vi "SetSocketOption.vi"(7 "path override":path, 8 "error in":errorcluster, 9 "value":variant, 10 "Socket option":T1=enum."ZMQ_SWAP", 11 "socket in":u64) -> (0 "error out":errorcluster, 3 "socket out":u64)   [LabVIEW 2025, in "LibZMQ.lvlib"]
uses:
  LibZMQ.lvlib
  ctls/SocketOption.ctl
  errno.vi
  strerror.vi
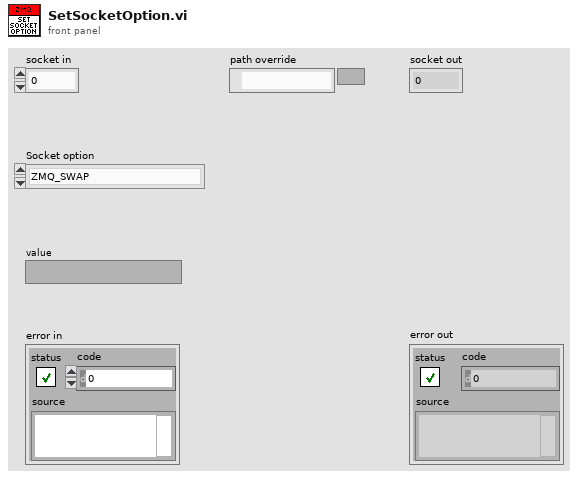
[diagram p1: front panel]
types:
  T1 = typedef "LibZMQ.lvlib/SocketOption.ctl" = enum8{"NONE", "ZMQ_HWM", "<2>", "ZMQ_SWAP", "ZMQ_AFFINITY", "ZMQ_ROUTING_ID", "ZMQ_SUBSCRIBE", "ZMQ_UNSUBSCRIBE", "ZMQ_RATE", "ZMQ_RECOVERY_IVL", "ZMQ_MCAST_LOOP", "ZMQ_SNDBUF", "ZMQ_RCVBUF", "ZMQ_RCVMORE", "ZMQ_FD", "ZMQ_EVENTS", "ZMQ_TYPE", "ZMQ_LINGER", "ZMQ_RECONNECT_IVL", "ZMQ_BACKLOG", "ZMQ_RECOVERY_IVL_MSEC", "ZMQ_RECONNECT_IVL_MAX", "ZMQ_MAXMSGSIZE", "ZMQ_SNDHWM", "ZMQ_RCVHWM", "ZMQ_MULTICAST_HOPS", "<26>", "ZMQ_RCVTIMEO", "ZMQ_SNDTIMEO", "<29>", "<30>", "ZMQ_IPV4ONLY", "ZMQ_LAST_ENDPOINT", "ZMQ_ROUTER_MANDATORY", "ZMQ_TCP_KEEPALIVE", "ZMQ_TCP_KEEPALIVE_CNT", "ZMQ_TCP_KEEPALIVE_IDLE", "ZMQ_TCP_KEEPALIVE_INTVL", "ZMQ_TCP_ACCEPT_FILTER", "ZMQ_IMMEDIATE", "ZMQ_XPUB_VERBOSE", "ZMQ_ROUTER_RAW", "ZMQ_IPV6", "ZMQ_MECHANISM", "ZMQ_PLAIN_SERVER", "ZMQ_PLAIN_USERNAME", "ZMQ_PLAIN_PASSWORD", "ZMQ_CURVE_SERVER", "ZMQ_CURVE_PUBLICKEY", "ZMQ_CURVE_SECRETKEY", "ZMQ_CURVE_SERVERKEY", "ZMQ_PROBE_ROUTER", "ZMQ_REQ_CORRELATE", "ZMQ_REQ_RELAXED", "ZMQ_CONFLATE", "ZMQ_ZAP_DOMAIN", "ZMQ_ROUTER_HANDOVER", "ZMQ_TOS", "ZMQ_IPC_FILTER_PID", "ZMQ_IPC_FILTER_UID", "ZMQ_IPC_FILTER_GID", "ZMQ_CONNECT_ROUTING_ID", "ZMQ_GSSAPI_SERVER", "ZMQ_GSSAPI_PRINCIPAL", "ZMQ_GSSAPI_SERVICE_PRINCIPAL", "ZMQ_GSSAPI_PLAINTEXT", "ZMQ_HANDSHAKE_IVL", "<67>", "ZMQ_SOCKS_PROXY", "ZMQ_XPUB_NODROP", "ZMQ_BLOCKY", "ZMQ_XPUB_MANUAL", "ZMQ_XPUB_WELCOME_MSG", "ZMQ_STREAM_NOTIFY", "ZMQ_INVERT_MATCHING", "ZMQ_HEARTBEAT_IVL", "ZMQ_HEARTBEAT_TTL", "ZMQ_HEARTBEAT_TIMEOUT", "ZMQ_XPUB_VERBOSER", "ZMQ_CONNECT_TIMEOUT", "ZMQ_TCP_MAXRT", "ZMQ_THREAD_SAFE", "<82>", "<83>", "ZMQ_MULTICAST_MAXTPDU", "ZMQ_VMCI_BUFFER_SIZE", "ZMQ_VMCI_BUFFER_MIN_SIZE", "ZMQ_VMCI_BUFFER_MAX_SIZE", "ZMQ_VMCI_CONNECT_TIMEOUT", "ZMQ_USE_FD", "ZMQ_GSSAPI_PRINCIPAL_NAMETYPE", "ZMQ_GSSAPI_SERVICE_PRINCIPAL_NAMETYPE", "ZMQ_BINDTODEVICE", "ZMQ_ZAP_ENFORCE_DOMAIN", "ZMQ_LOOPBACK_FASTPATH", "ZMQ_METADATA", "ZMQ_MULTICAST_LOOP", "ZMQ_ROUTER_NOTIFY"}
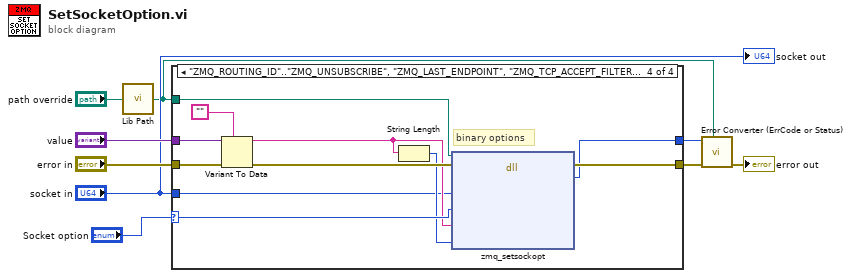
[diagram p0: block diagram]
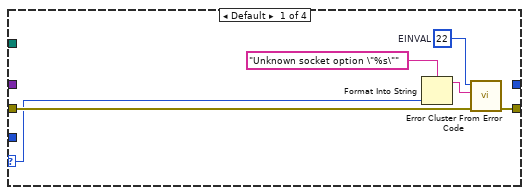
[diagram p2: hidden frame]
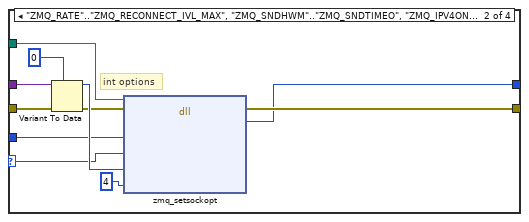
[diagram p3: hidden frame]
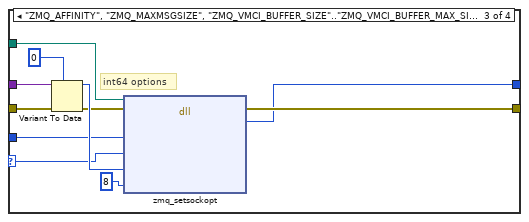
[diagram p4: hidden frame]
diagram:
  n1 = call "Lib Path.vi"("path override"="path override") -> ("lib path"=w1:path)
  n2 = case shown="\"ZMQ_ROUTING_ID\"..\"ZMQ_UNSUBSCRIBE\", \"ZMQ_LAST_ENDPOINT\", \"ZMQ_TCP_ACCEPT_FILTER\", \"ZMQ_PLAIN_USERNAME\", \"ZMQ_PLAIN_PASSWORD\", \"ZMQ_CURVE_PUBLICKEY\"..\"ZMQ_CURVE_SERVERKEY\", \"ZMQ_ZAP_DOMAIN\", \"ZMQ_CONNECT_ROUTING_ID\", \"ZMQ_GSSAPI_PRINCIPAL\", \"ZMQ_GSSAPI_SERVICE_PRINCIPAL\", \"ZMQ_SOCKS_PROXY\", \"ZMQ_XPUB_WELCOME_MSG\", \"ZMQ_BINDTODEVICE\", \"ZMQ_METADATA\"" "Socket option" {
    selector: "Socket option" -> [w12 w19 w30 w42]
    tunnel: [w15 w26 w37 w48] -> w5
    tunnel: [_ w25 w36 w47] -> w6
    tunnel: "value" -> [_ w24 w35 w46]
    tunnel: "error in" -> [w13 w21 w32 w44]
    tunnel: w1 -> [_ w17 w28 w39]
    tunnel: "socket in" -> [_ w16 w27 w38]
    frame Default {
      w14 = 22  # EINVAL
      n3 = Format Into String(format string="Unknown socket option \"%s\"", w12) -> (resulting string=w10:string)  [unwired: 2 in, 1 out]
      n4 = call <vilib>:"Error Cluster From Error Code.vi"("error in (no error)"=w13, "error message (\"\")"=w10, "error code (0)"=w14) -> ("error out"=w15:errorcluster)  [unwired: 6 in]
    }
    frame "ZMQ_RATE".."ZMQ_RECONNECT_IVL_MAX", "ZMQ_SNDHWM".."ZMQ_SNDTIMEO", "ZMQ_IPV4ONLY", "ZMQ_ROUTER_MANDATORY".."ZMQ_TCP_KEEPALIVE_INTVL", "ZMQ_IMMEDIATE".."ZMQ_IPV6", "ZMQ_PLAIN_SERVER", "ZMQ_CURVE_SERVER", "ZMQ_PROBE_ROUTER".."ZMQ_CONFLATE", "ZMQ_ROUTER_HANDOVER", "ZMQ_TOS", "ZMQ_GSSAPI_SERVER", "ZMQ_GSSAPI_PLAINTEXT", "ZMQ_HANDSHAKE_IVL", "ZMQ_XPUB_NODROP", "ZMQ_XPUB_MANUAL", "ZMQ_STREAM_NOTIFY".."ZMQ_TCP_MAXRT", "ZMQ_MULTICAST_MAXTPDU", "ZMQ_VMCI_CONNECT_TIMEOUT".."ZMQ_GSSAPI_SERVICE_PRINCIPAL_NAMETYPE", "ZMQ_ZAP_ENFORCE_DOMAIN", "ZMQ_MULTICAST_LOOP", "ZMQ_ROUTER_NOTIFY" {
      # "int options"
      n5 = Variant To Data(error in=w21, type=0, Variant=w24) -> (data=w23:i32, error out=w20:errorcluster)
      n6 = dll-call lib="C:/git/ZMQLV/libzmq-v143-mt-4_3_6/lib/win32/libzmq-v143-mt-4_3_6.dll" fn="zmq_setsockopt" ("zmq_labview.dll:lvzmq_setsockopt")(path in=w17, error in=w20, "socket"=w16, "option"=w19, "data"=w23, "len"=u32 4) -> (error out=w26:errorcluster, "return type"=w25:i32)  [unwired: 5 in, 1 out]
    }
    frame "ZMQ_AFFINITY", "ZMQ_MAXMSGSIZE", "ZMQ_VMCI_BUFFER_SIZE".."ZMQ_VMCI_BUFFER_MAX_SIZE" {
      # "int64 options"
      n7 = Variant To Data(error in=w32, type=i64 0, Variant=w35) -> (data=w34:i64, error out=w31:errorcluster)
      n8 = dll-call lib="C:/git/ZMQLV/libzmq-v143-mt-4_3_6/lib/win32/libzmq-v143-mt-4_3_6.dll" fn="zmq_setsockopt" ("zmq_labview.dll:lvzmq_setsockopt")(path in=w28, error in=w31, "socket"=w27, "option"=w30, "data"=w34, "len"=u32 8) -> (error out=w37:errorcluster, "return type"=w36:i32)  [unwired: 5 in, 1 out]
    }
    frame "ZMQ_ROUTING_ID".."ZMQ_UNSUBSCRIBE", "ZMQ_LAST_ENDPOINT", "ZMQ_TCP_ACCEPT_FILTER", "ZMQ_PLAIN_USERNAME", "ZMQ_PLAIN_PASSWORD", "ZMQ_CURVE_PUBLICKEY".."ZMQ_CURVE_SERVERKEY", "ZMQ_ZAP_DOMAIN", "ZMQ_CONNECT_ROUTING_ID", "ZMQ_GSSAPI_PRINCIPAL", "ZMQ_GSSAPI_SERVICE_PRINCIPAL", "ZMQ_SOCKS_PROXY", "ZMQ_XPUB_WELCOME_MSG", "ZMQ_BINDTODEVICE", "ZMQ_METADATA" {
      # "binary options"
      n9 = Variant To Data(error in=w44, type="", Variant=w46) -> (data=w40:string, error out=w43:errorcluster)
      n10 = String Length(string=w40) -> (length=w41:i32)
      n11 = dll-call lib="C:/git/ZMQLV/libzmq-v143-mt-4_3_6/lib/win32/libzmq-v143-mt-4_3_6.dll" fn="zmq_setsockopt" ("zmq_labview.dll:lvzmq_setsockopt")(path in=w39, error in=w43, "socket"=w38, "option"=w42, "data"=w40, "len"=w41) -> (error out=w48:errorcluster, "return type"=w47:i32)  [unwired: 5 in, 1 out]
    }
  }
  n12 = call "Error Converter (ErrCode or Status).vi"("path override"=w1, "error in (no error)"=w5, "error code"=w6) -> ("error out"=→"error out":errorcluster)  [unwired: 8 in]
  "socket out" <- "socket in"
